vi "Stage position FGV.vi"(10 "Stage status (in)":T1, 11 "Action":enum16{"read", "write", "clear"}(ring)) -> (2 "Stage status (out)":T1)   [LabVIEW 2020]
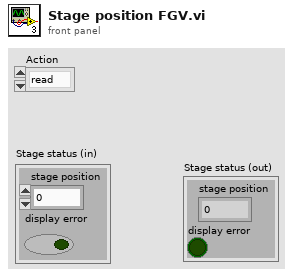
[diagram p1: front panel]
types:
  T1 = cluster{"stage position":dbl, "display error":bool}
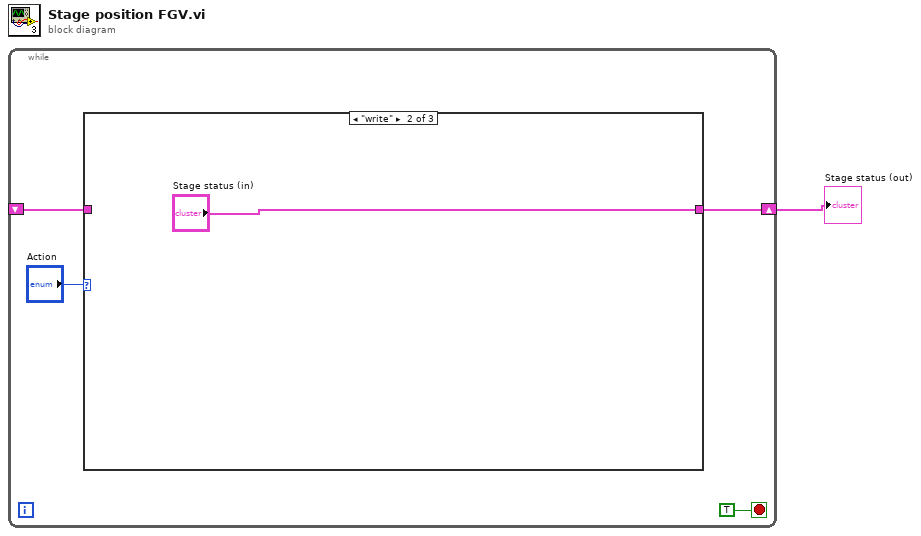
[diagram p0: block diagram]
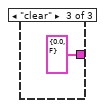
[diagram p3: hidden frame]
diagram:
  n1 = while {
    shift-right: [w3] -> w1
    shift-left: _ -> [w2]
    stop <- TRUE stop-if-true
    n2 = case shown="\"write\"" "Action" {
      tunnel: [w6 "Stage status (in)" T1 {"stage position"=0.0, "display error"=FALSE} ("Stage status")] -> w3
      tunnel: w2 -> [w6 _ _]
      frame "read", Default {
      }
      frame "write" {
      }
      frame "clear" {
      }
    }
  }
  "Stage status (out)" <- w1
